vi "Read Saved Taus.vi"() -> ()   [LabVIEW 2014]
panel:
  out "Waveform Graph 2":dbl[](graph)
  out "size(s)":dbl
  out "Array":timestamp[](array[timestamp])
  out "Waveform Graph":dbl[](graph)
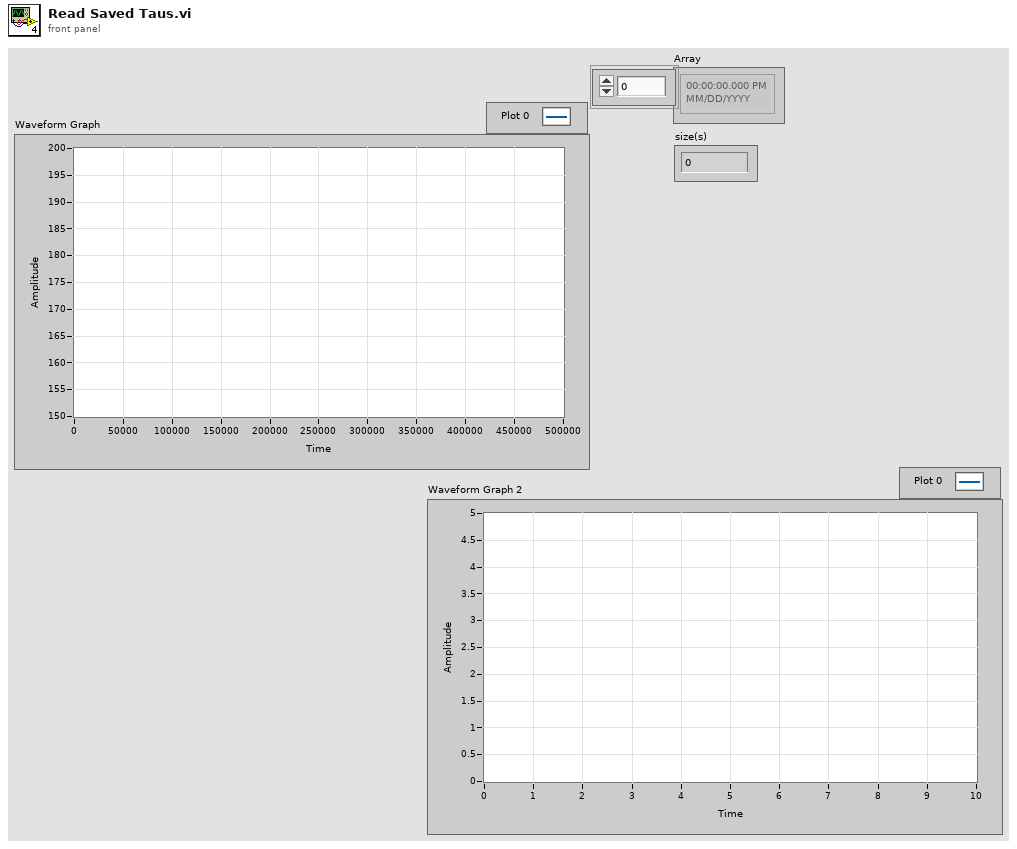
[diagram p1: front panel]
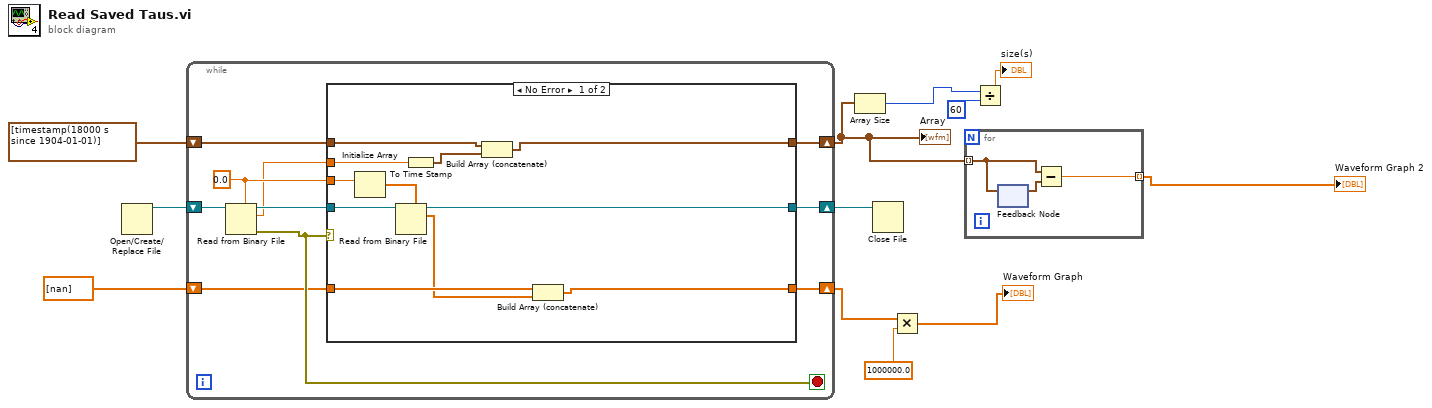
[diagram p0: block diagram]
diagram:
  n1 = Open/Create/Replace File() -> (refnum out=w9:refnum<file>)  [unwired: 6 in, 2 out]
  n2 = while {
    shift-right: [w20] -> w11
    shift-left: w9 -> [w22]
    shift-right: [w15] -> w2
    shift-left: timestamp[] [timestamp(18000 s since 1904-01-01)] -> [w17]
    shift-right: [w13] -> w6
    shift-left: dbl[] [nan] -> [w14]
    stop <- w19 stop-if-true
    w18 = 0.0
    n3 = Read from Binary File(5:w18, 11:w22) -> (0:w19:errorcluster, 2:w16:dbl, 3:w21:refnum<file>)  [unwired: 4 in, 1 out]
    n4 = case shown="No Error" w19 {
      tunnel: w21 -> [w33 w35]
      tunnel: [w32 w35] -> w20
      tunnel: w18 -> [w31 _]
      tunnel: w17 -> [w27 w36]
      tunnel: w16 -> [w29 _]
      tunnel: [w26 w36] -> w15
      tunnel: w14 -> [w25 w34]
      tunnel: [w23 w34] -> w13
      frame No Error {
        n5 = Initialize Array(w31) -> (w30:dbl[])  [unwired: 1 in]
        n6 = Read from Binary File(5:w30, 11:w33) -> (2:w24:dbl[], 3:w32:refnum<file>)  [unwired: 4 in, 2 out]
        n7 = To Time Stamp(1:w29) -> (0:w28:timestamp)
        n8 = Build Array (concatenate)(w27, w28) -> (w26:timestamp[])
        n9 = Build Array (concatenate)(w25, w24) -> (w23:dbl[])
      }
      frame Error {
      }
    }
  }
  "Array" <- w2
  n10 = Array Size(array=w2) -> (size(s)=w5:i32)
  n11 = Close File(refnum=w11) -> ()  [unwired: 1 in, 2 out]
  n12 = Multiply(x=w6, y=1000000.0) -> (x*y=→"Waveform Graph":dbl[])
  n13 = for {
    tunnel: w2 -> [w39] mode=indexing
    tunnel: [w37] -> w1 mode=indexing
    n14 = feedback-in #1(w39) -> ()
    n15 = feedback #1() -> (w38:timestamp)  [unwired: 1 in]
    n16 = Subtract(x=w39, y=w38) -> (x-y=w37:dbl)
  }
  "Waveform Graph 2" <- w1
  n17 = Divide(x=w5, y=60) -> (x/y=→"size(s)":dbl)
